vi "- VI Tree - JKI JSON Serialization.vi"   [LabVIEW 2020]
uses:
  <userlib>/_OpenG.lib/lvdata/lvdata.llb/Array Size(s)__ogtk.vi
  <userlib>/_OpenG.lib/lvdata/lvdata.llb/Array of VData to VCluster__ogtk.vi
  JKI JSON Serialization.lvlib
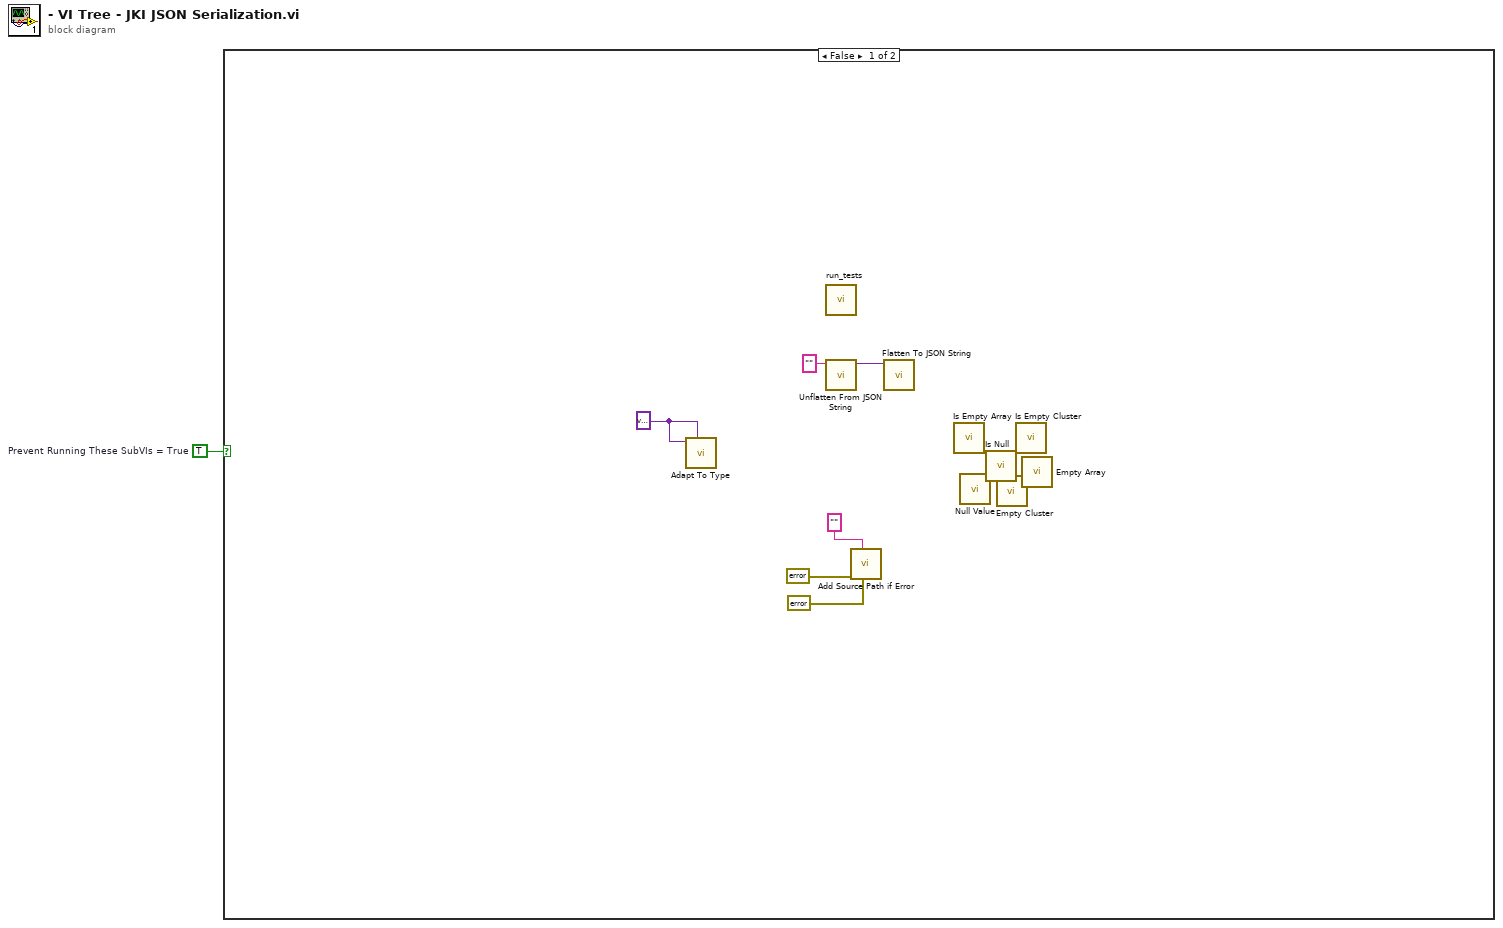
[diagram p0: block diagram]
diagram:
  w1 = TRUE  # Prevent Running These SubVIs = True
  n1 = case shown="False" w1 {
    frame False {
      w2 = variant ("Type and Defaults")
      n2 = call "Adapt To Type.vi"("Type and Defaults"=w2, "Variant in"=w2) -> ()  [unwired: 8 in, 2 out]
      n3 = call "run_tests.vi"() -> ()  [unwired: 12 in]
      n4 = call "Unflatten From JSON String.vi"("JSON String"="") -> ("Variant"=w7:variant)  [unwired: 9 in, 1 out]
      n5 = call "Add Source Path if Error.vi"("Upstream Error"=errorcluster {"status"=FALSE, "code"=0, "source"=""} ("error in"), "Source Path or URL"="", "error in"=errorcluster {"status"=FALSE, "code"=0, "source"=""}) -> ()  [unwired: 8 in, 1 out]
      n6 = call "Flatten To JSON String.vi"("Variant"=w7) -> ()  [unwired: 9 in, 2 out]
      n7 = call "Is Empty Array.vi"() -> ()  [unwired: 1 in, 1 out]
      n8 = call "Null Value.vi"() -> ()  [unwired: 1 out]
      n9 = call "Is Null.vi"() -> ()  [unwired: 1 in, 1 out]
      n10 = call "Empty Cluster.vi"() -> ()  [unwired: 1 out]
      n11 = call "Is Empty Cluster.vi"() -> ()  [unwired: 1 in, 1 out]
      n12 = call "Empty Array.vi"() -> ()  [unwired: 1 out]
    }
    frame True {
    }
  }
